vi "example_microFPGA_Servo.vi"() -> ()   [LabVIEW 2021]
panel:
  out "Servo_position_READ":u32(slide)=12706 max=65535 step=1 scale=0.0..65535.0 scale format="%u us"
  in  "Servo_channel":u16(ring) items=["channel No 0", "channel No 1", "channel No 2", "channel No 3", "channel No 4", "channel No 5", "channel No 6"]
  in  "write or read":u16(ring)=1 items=["read", "write"]
  out "value write confirm 5":bool
  in  "Servo_position_WRITE":u32(slide)=12706 max=65535 step=1 scale=0.0..65535.0 scale format="%u us"
  out "Version":u16=3
  in  "close Application":bool=TRUE
  in  "send parameters":bool
  # "Servo control"
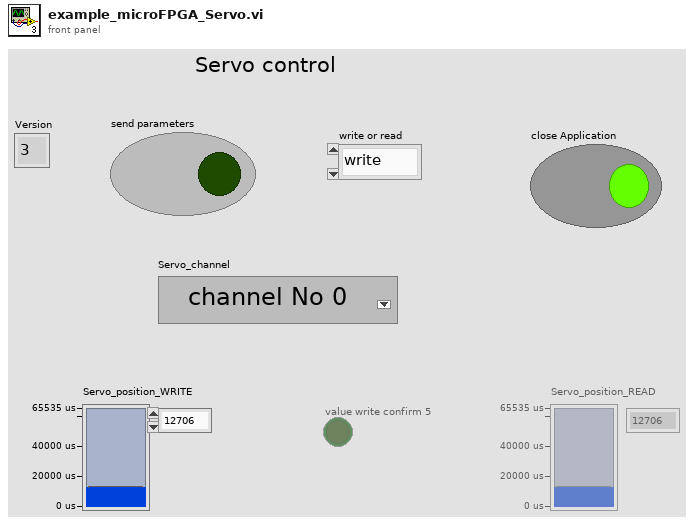
[diagram p1: front panel]
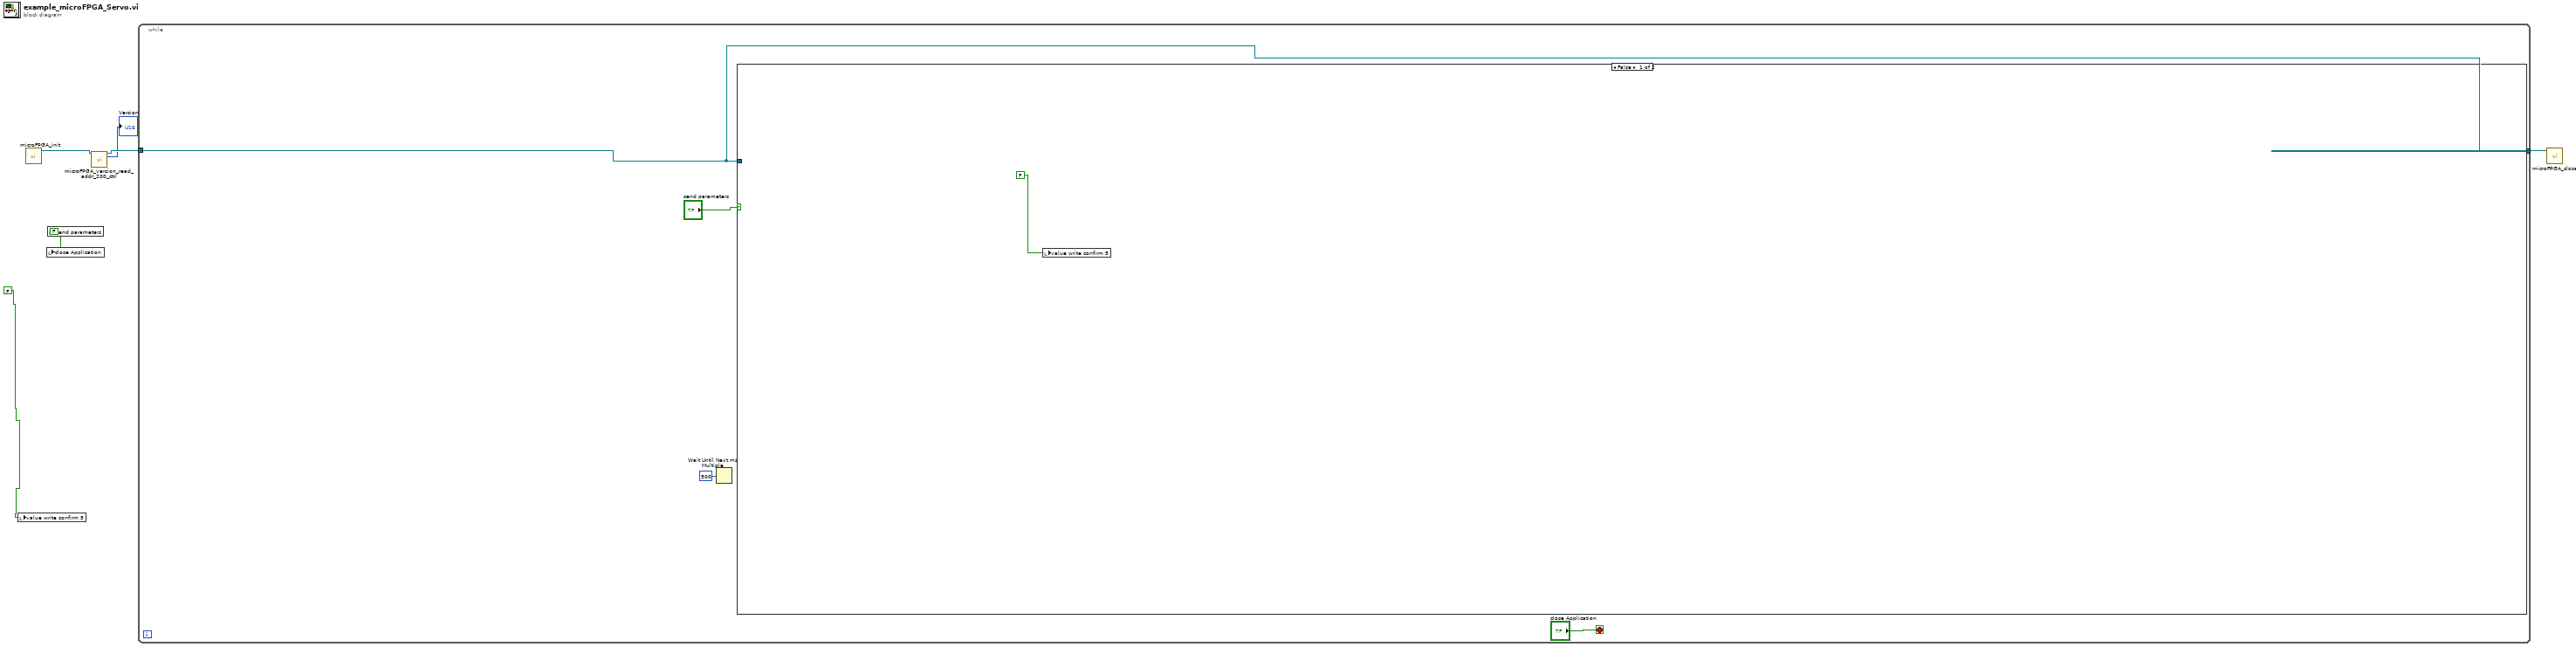
[diagram p0: block diagram]
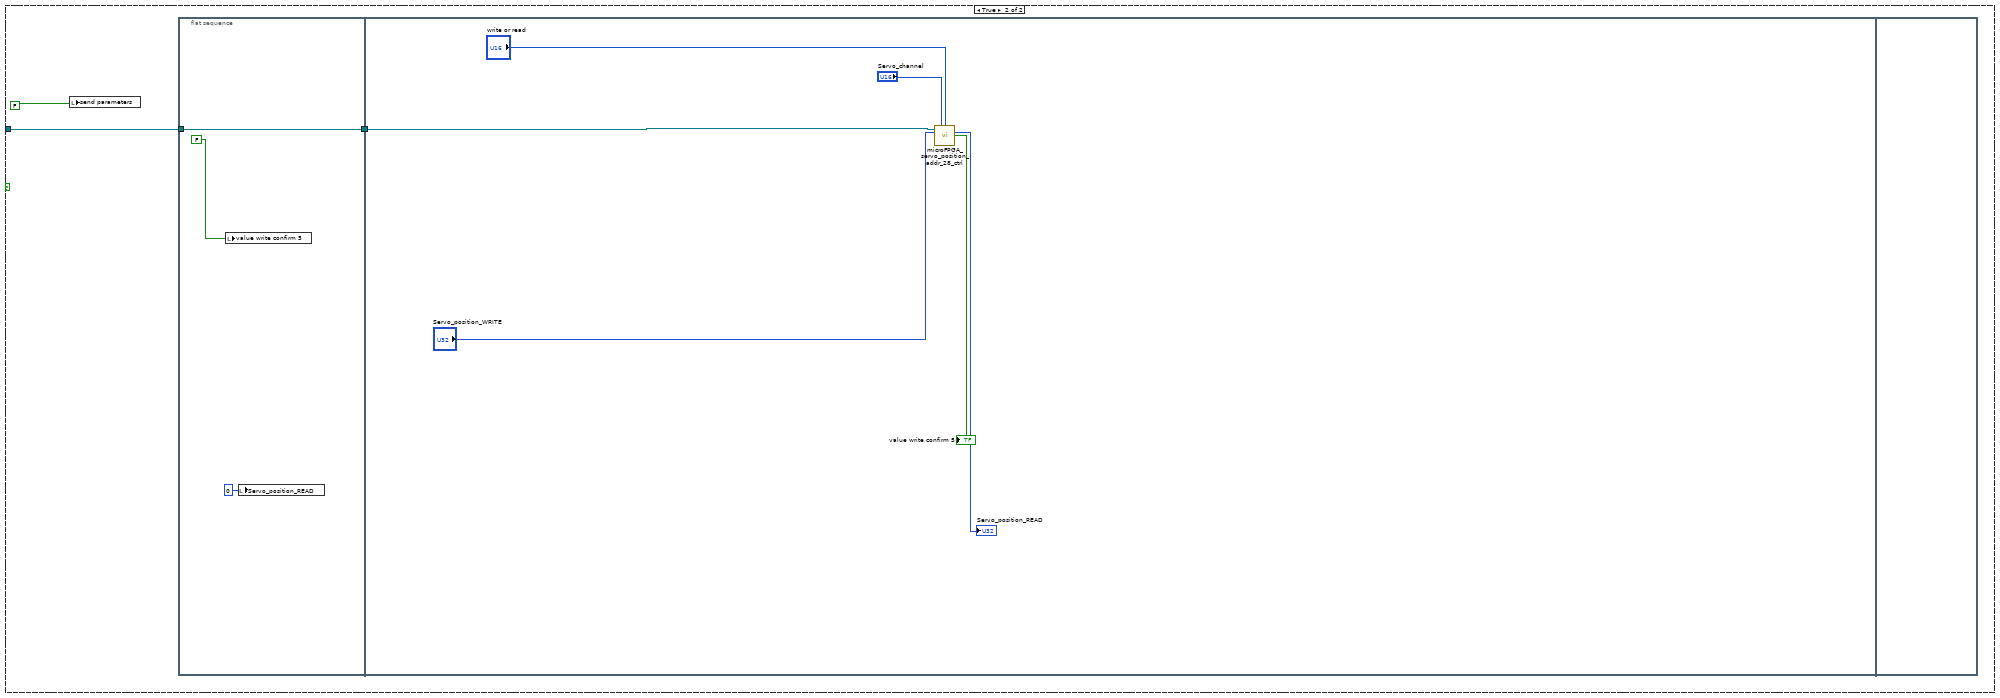
[diagram p2: hidden frame]
diagram:
  w6 = FALSE ("write")
  n1 = local write "value write confirm 5"(FALSE ("write")) -> ()
  n2 = call "microFPGA_init.vi"() -> ("VISA resource name out"=w4:refnum<visa-resource-name>)  [unwired: 10 in, 1 out]
  n3 = local write "close Application"(w6) -> ()
  n4 = local write "send parameters"(w6) -> ()
  n5 = call "microFPGA_version_read_addr_200_ctrl.vi"("VISA resource name"=w4) -> ("VISA resource name 2"=w3:refnum<visa-resource-name>, "Version"=→"Version":u16)  [unwired: 12 in, 1 out]
  n6 = while {
    tunnel: w3 -> [w7]
    tunnel: [w7] -> w5
    stop <- "close Application" stop-if-true
    n7 = Wait Until Next ms Multiple(millisecond multiple=u32 500) -> ()  [unwired: 1 out]
    n8 = case shown="False" "send parameters" {
      tunnel: w7 -> [_ w13]
      frame False {
        n9 = local write "value write confirm 5"(FALSE ("value write confirm")) -> ()
      }
      frame True {
        n10 = local write "send parameters"(FALSE ("write")) -> ()
        n11 = flat-sequence {
          tunnel: w13 -> [w17]
          tunnel: [w17] -> w12
          tunnel: w12 -> [w18]
          frame #0 {
            n12 = local write "value write confirm 5"(FALSE ("value write confirm")) -> ()
            n13 = local write "Servo_position_READ"(u32 0 ("Servo_position_READ")) -> ()
          }
          frame #1 {
            n14 = call "microFPGA_servo_position_addr_28_ctrl.vi"("VISA resource name"=w18, "Servo_channel"="Servo_channel", "write or read"="write or read", "Servo_position_WRITE"="Servo_position_WRITE") -> ("Servo_position_READ"=→"Servo_position_READ":u32, "value write confirm"=→"value write confirm 5":bool)  [unwired: 7 in, 3 out]
          }
          frame #2 {
          }
        }
      }
    }
  }
  n15 = call "microFPGA_close.vi"("VISA resource name"=w5) -> ()  [unwired: 11 in]
